vi "light_pose.vi"(11 "Point selector":T1={"Pose mode"=enum."Light", "Light number"=5} {"Light number" min=0 max=5}) -> (3 "Light pose (ASAP coordinates)":T2)   [LabVIEW 2013]
uses:
  <vilib>/Analysis/Matrix/Datatypes/RealMatrix.ctl
  calibration/point_selector.ctl
  calibration/array_3d_double.ctl
  <vilib>/Analysis/Matrix/NI_Matrix.lvlib
panel:
  # "Return pose centered on specified light in \"Light\" mode, or either pose estimate."
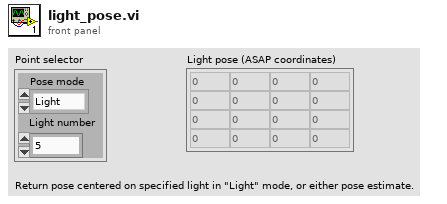
[diagram p1: front panel]
types:
  T1 = typedef "point_selector.ctl" = cluster{"Pose mode":enum16{"Light", "Handle", "Output"}, "Light number":i32}
  T2 = typedef "NI_Matrix.lvlib/RealMatrix.ctl" = dbl[][]
  T3 = typedef "array_3d_double.ctl" = dbl[][][]
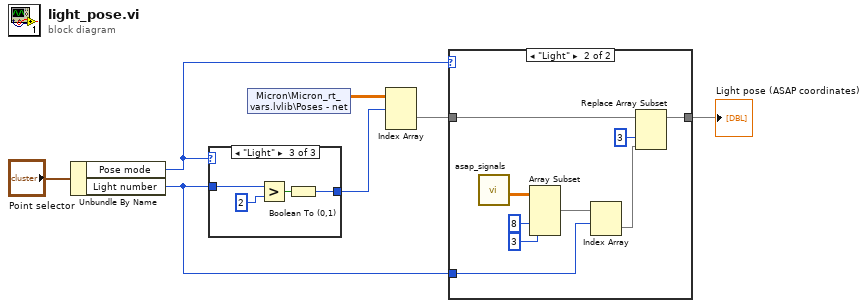
[diagram p0: block diagram]
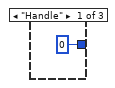
[diagram p2: hidden frame]
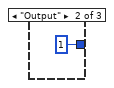
[diagram p3: hidden frame]
diagram:
  n1 = Unbundle By Name("Point selector") -> ("Pose mode"=w3:enum16{"Light", "Handle", "Output"}, "Light number"=w2:i32)
  n2 = case shown="\"Light\"" w3 {
    tunnel: w2 -> [_ _ w13]
    tunnel: [i16 0 i16 1 w11] -> w5
    frame "Handle" {
    }
    frame "Output" {
    }
    frame "Light" {
      n3 = Greater?(x=w13, y=2) -> (0:w10:bool)
      n4 = Boolean To (0,1)(Boolean=w10) -> (0, 1=w11:i16)
    }
  }
  n5 = shared-variable "Micron\\Micron_rt_vars.lvlib\\Poses - net"() -> (w6:T3)  [unwired: 1 in, 1 out]
  n6 = Index Array(array=w6, index (dim 0)=w5) -> (element=w1:dbl[][])  [unwired: 2 in]
  n7 = case shown="\"Light\"" w3 {
    tunnel: [w14 w23] -> w7
    tunnel: w1 -> [w14 w20]
    tunnel: w2 -> [_ w15]
    frame Default {
    }
    frame "Light" {
      n8 = call "asap_signals.vi"() -> ("ASAP signals"=w18:sgl[][])  [unwired: 10 in, 1 out]
      n9 = Array Subset(array=w18, index (col)=8 ("length"), length (col)=3 ("length")) -> (w16:sgl[][])  [unwired: 2 in]
      n10 = Index Array(array=w16, index (row)=w15) -> (element=w22:sgl[])  [unwired: 1 in]
      n11 = Replace Array Subset(array=w20, new element=w22, index (col)=3 ("disabled index (col)")) -> (w23:dbl[][])  [unwired: 1 in]
    }
  }
  "Light pose (ASAP coordinates)" <- w7
